vi "student_toeplitz 1.vi"(4 "error in (no error)":errorcluster, 6 "column":cdb[](array[numeric]), 7 "row":cdb[](array[numeric])) -> (0 "error out":errorcluster, 3 "Toeplitz Array":cdb[][](array[numeric]))   [LabVIEW 2013]
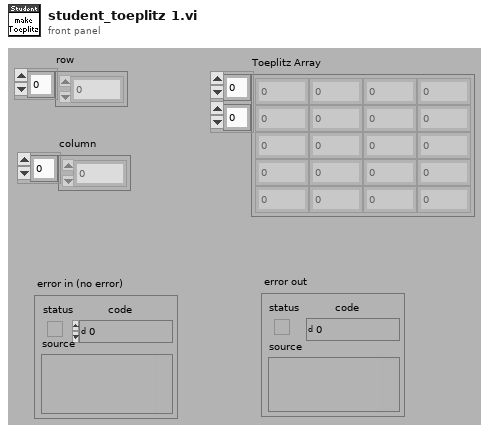
[diagram p1: front panel]
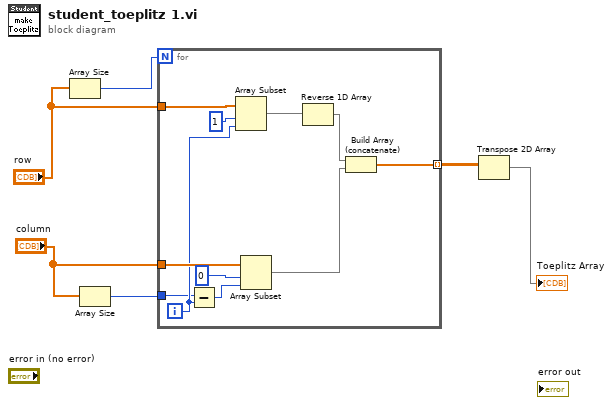
[diagram p0: block diagram]
diagram:
  n1 = Array Size(array="row") -> (size(s)=w6:i32)
  n2 = Array Size(array="column") -> (size(s)=w3:i32)
  n3 = for {
    N: w6 -> [_]
    tunnel: "row" -> [w16]
    tunnel: "column" -> [w15]
    tunnel: w3 -> [w12]
    tunnel: [w7] -> w2 mode=indexing
    i -> [w13]
    n4 = Subtract(x=w12, y=w13) -> (x-y=w11:i32)
    n5 = Array Subset(array=w16, index=1, length=w13) -> (w10:cdb[])
    n6 = Array Subset(array=w15, index=0, length=w11) -> (w8:cdb[])
    n7 = Reverse 1D Array(array=w10) -> (reversed array=w9:cdb[])
    n8 = Build Array (concatenate)(w9, w8) -> (w7:cdb[])
  }
  n9 = Transpose 2D Array(2D array=w2) -> (transposed array=→"Toeplitz Array":cdb[][])
